vi "GCMPlugin_GetPluginName.vi"(8 "error in (no error)":errorcluster, 11 "_BasicVIDocumentation in":refnum<class "BasicClassDocumentation.lvclass">) -> (0 "error out":errorcluster, 2 "PluginName":string, 3 "_BasicVIDocumentation out":refnum<class "BasicClassDocumentation.lvclass">)   [LabVIEW 2014, in "BasicClassDocumentation.lvlib" / "BasicClassDocumentation.lvclass"]
uses:
  BasicClassDocumentation.lvclass
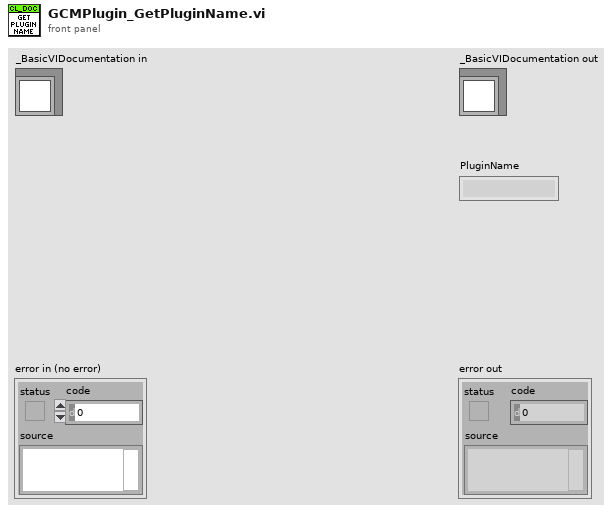
[diagram p1: front panel]
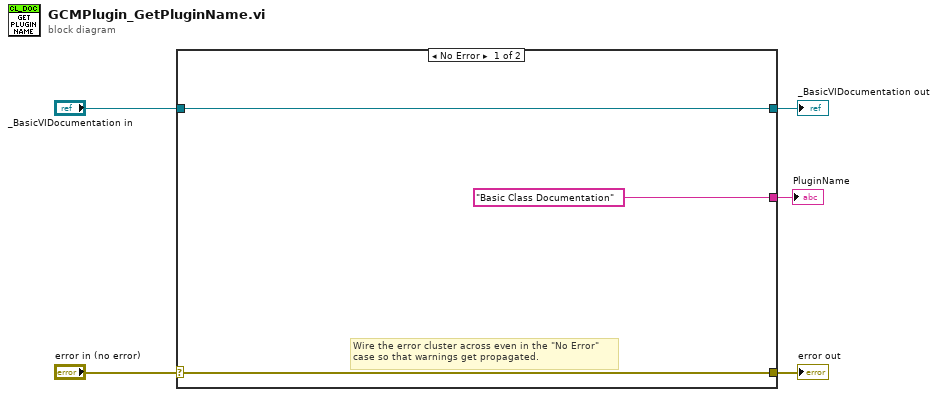
[diagram p0: block diagram]
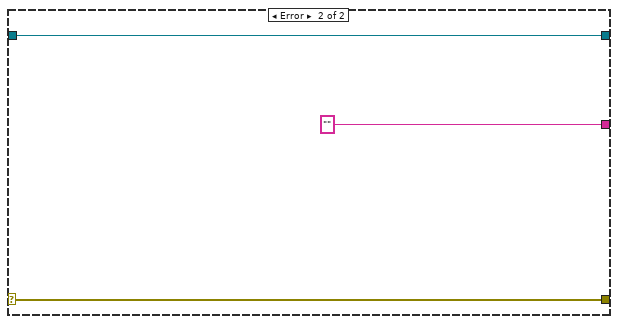
[diagram p2: hidden frame]
diagram:
  n1 = case shown="No Error" "error in (no error)" {
    selector: "error in (no error)" -> [w7 w11]
    tunnel: [w7 w11] -> w4
    tunnel: [w8 w10] -> w2
    tunnel: "_BasicVIDocumentation in" -> [w8 w10]
    tunnel: ["Basic Class Documentation" ""] -> w1
    frame No Error {
      # "Wire the error cluster across even in the \"No Error\"\ncase so that warnings get propagated."
    }
    frame Error {
    }
  }
  "error out" <- w4
  "_BasicVIDocumentation out" <- w2
  "PluginName" <- w1
